vi "Use Current Time If Empty.vi"(3 "Time(Empty to Use Current Time)":timestamp) -> (1 "Time out":timestamp)   [LabVIEW 2017]
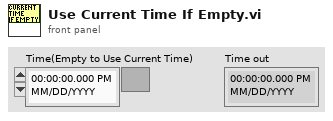
[diagram p1: front panel]
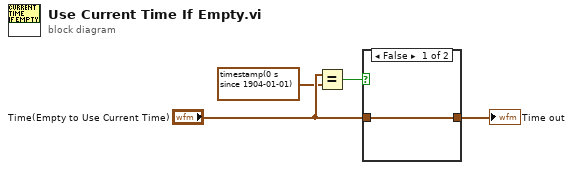
[diagram p0: block diagram]
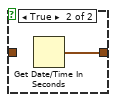
[diagram p2: hidden frame]
diagram:
  n1 = Equal?(x="Time(Empty to Use Current Time)", y=timestamp(0 s since 1904-01-01) ("seconds since 1Jan1904")) -> (x = y?=w2:bool)
  n2 = case shown="False" w2 {
    tunnel: [w5 w6] -> w4
    tunnel: "Time(Empty to Use Current Time)" -> [w5 _]
    frame False {
    }
    frame True {
      n3 = Get Date/Time In Seconds() -> (seconds since 1Jan1904=w6:timestamp)
    }
  }
  "Time out" <- w4
